vi "XY Graph Get Plot Info & Clip Data.vi"(8 "error in (no error)":errorcluster, 9 "Clip Plot? (True)":bool=TRUE, 10 "Plot index":i32, 11 "XYGraph Ref in":refnum<vi>) -> (0 "error out":errorcluster, 1 "Y Array":dbl[](array[numeric]), 2 "X Array":dbl[](array[numeric]), 3 "XYGraph Ref out":refnum<vi>, 4 "Plot Name":string, 5 "Plot Range":T1, 6 "Plot Color":u32, 7 "Plot Clipped?":bool)   [LabVIEW 2021, in "XY Graph Add-Ons.lvlib"]
doc: "Returns the <B>X</B> and <B>Y</B> array of the selected plot and optionally removes points which are not visible in the <B>XY Graph</B>."
uses:
  XY Graph Add-Ons.lvlib
  Plot Range.ctl
  Graphs.lvlib
panel:
  # "-1: last plot\n-2: next to last plot\n-3: etc..."
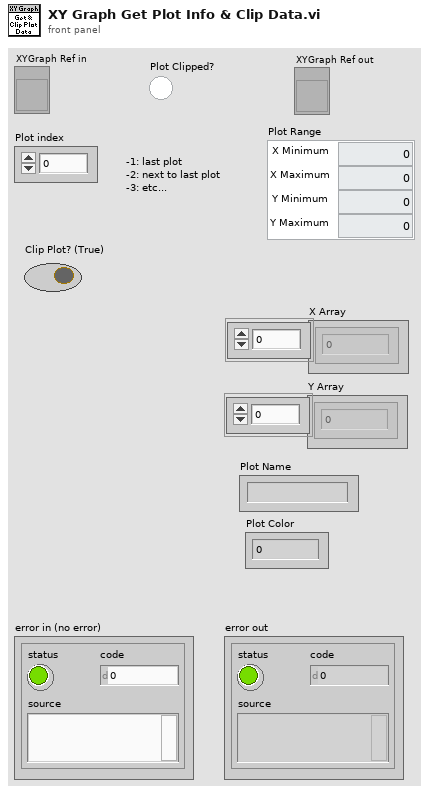
[diagram p1: front panel]
types:
  T1 = typedef "Graphs.lvlib/Plot Range.ctl" = cluster{"X Minimum":dbl, "X Maximum":dbl, "Y Minimum":dbl, "Y Maximum":dbl}
  T2 = cluster{"X Array out":dbl[], "Y Array out":dbl[]}
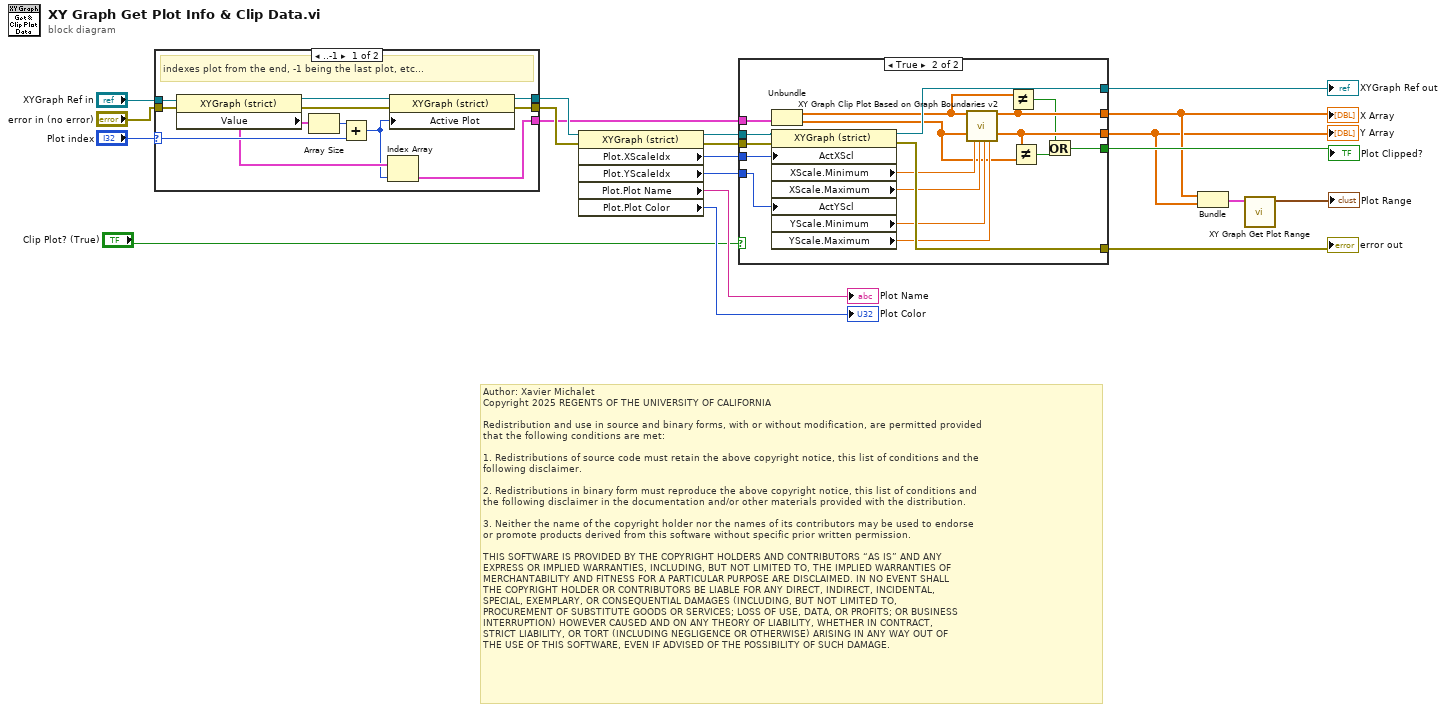
[diagram p0: block diagram]
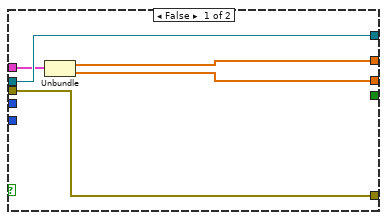
[diagram p2: hidden frame]
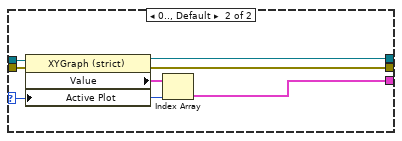
[diagram p3: hidden frame]
diagram:
  # "Author: Xavier Michalet\nCopyright 2025 REGENTS OF THE UNIVERSITY OF CALIFORNIA\n\nRedistribution and use in source and binary forms, with or without modification, are permitted provided\nthat the following conditions are met:\n\n1. Redistributions of source code must retain the above copyright notice, this list of conditions and the\nfollowing disclaimer.\n\n2. Redistributions in binary form must reproduce the above copyright notice, this list of conditions and\nthe following disclaimer in the documentation and/or other materials provided with the distribution.\n\n3. Neither the name of the copyright holder nor the names of its contributors may be used to endorse \nor promote products derived from this software without specific prior written permission.\n\nTHIS SOFTWARE IS PROVIDED BY THE COPYRIGHT HOLDERS AND CONTRIBUTORS “AS IS” AND ANY \nEXPRESS OR IMPLIED WARRANTIES, INCLUDING, BUT NOT LIMITED TO, THE IMPLIED WARRANTIES OF\nMERCHANTABILITY AND FITNESS FOR A PARTICULAR PURPOSE ARE DISCLAIMED. IN NO EVENT SHALL\nTHE COPYRIGHT HOLDER OR CONTRIBUTORS BE LIABLE FOR ANY DIRECT, INDIRECT, INCIDENTAL, \nSPECIAL, EXEMPLARY, OR CONSEQUENTIAL DAMAGES (INCLUDING, BUT NOT LIMITED TO, \nPROCUREMENT OF SUBSTITUTE GOODS OR SERVICES; LOSS OF USE, DATA, OR PROFITS; OR BUSINESS\nINTERRUPTION) HOWEVER CAUSED AND ON ANY THEORY OF LIABILITY, WHETHER IN CONTRACT, \nSTRICT LIABILITY, OR TORT (INCLUDING NEGLIGENCE OR OTHERWISE) ARISING IN ANY WAY OUT OF\nTHE USE OF THIS SOFTWARE, EVEN IF ADVISED OF THE POSSIBILITY OF SUCH DAMAGE."
  n1 = case shown="..-1" "Plot index" {
    selector: "Plot index" -> [w28 w33]
    tunnel: [w25 w37] -> w11
    tunnel: "XYGraph Ref in" -> [w31 w36]
    tunnel: "error in (no error)" -> [w30 w35]
    tunnel: [w24 w34] -> w8
    tunnel: [w21 w32] -> w6
    frame ..-1 {
      # "indexes plot from the end, -1 being the last plot, etc..."
      n2 = property class="XYGraph (strict)"(reference=w31, error in=w30) -> (reference out=w27:refnum<vi>, error out=w26:errorcluster, "Value"=w23:cluster{dbl[], dbl[]}[])
      n3 = Array Size(array=w23) -> (size(s)=w29:i32)
      n4 = Add(x=w29, y=w28) -> (x+y=w22:i32)
      n5 = Index Array(array=w23, index=w22) -> (element=w21:cluster{dbl[], dbl[]})
      n6 = property class="XYGraph (strict)"(reference=w27, error in=w26, "Active Plot"=w22) -> (reference out=w25:refnum<vi>, error out=w24:errorcluster)
    }
    frame 0.., Default {
      n7 = property class="XYGraph (strict)"(reference=w36, error in=w35, "Active Plot"=w33) -> (reference out=w37:refnum<vi>, error out=w34:errorcluster, "Value"=w38:cluster{dbl[], dbl[]}[])
      n8 = Index Array(array=w38, index=w33) -> (element=w32:cluster{dbl[], dbl[]})
    }
  }
  n9 = property class="XYGraph (strict)"(reference=w11, error in=w8) -> (reference out=w17:refnum<vi>, error out=w15:errorcluster, "Plot.XScaleIdx"=w13:u32, "Plot.YScaleIdx"=w12:u32, "Plot.Plot Name"=→"Plot Name":string, "Plot.Plot Color"=→"Plot Color":u32)
  n10 = case shown="True" "Clip Plot? (True)" {
    tunnel: w6 -> [w41 w55]
    tunnel: w17 -> [w43 w61]
    tunnel: [w43 w59] -> w16
    tunnel: w15 -> [w42 w60]
    tunnel: [w42 w58] -> w14
    tunnel: w13 -> [_ w57]
    tunnel: w12 -> [_ w56]
    tunnel: [w40 w50] -> w3
    tunnel: [w39 w48] -> w2
    tunnel: [_ w44] -> w4
    frame False {
      n11 = Unbundle(w41) -> (w40:dbl[], w39:dbl[])
    }
    frame True {
      n12 = Unbundle(w55) -> (w49:dbl[], w47:dbl[])
      n13 = property class="XYGraph (strict)"(reference=w61, error in=w60, "ActXScl"=w57, "ActYScl"=w56) -> (reference out=w59:refnum<vi>, error out=w58:errorcluster, "XScale.Minimum"=w54:dbl, "XScale.Maximum"=w53:dbl, "YScale.Minimum"=w52:dbl, "YScale.Maximum"=w51:dbl)
      n14 = call "XY Graph Clip Plot Based on Graph Boundaries v2.vi"("X Array in"=w49, "Y Array in"=w47, "XScale.Minimum (-Inf)"=w54, "XScale.Maximum (Inf)"=w53, "YScale.Minimum (-Inf)"=w52, "YScale.Maximum (Inf)"=w51) -> ("X Array out"=w50:dbl[], "Y Array out"=w48:dbl[])  [unwired: 12 in]
      n15 = Not Equal?(x=w49, y=w50) -> (x != y?=w45:bool)
      n16 = Not Equal?(x=w48, y=w47) -> (x != y?=w46:bool)
      n17 = Or(x=w45, y=w46) -> (x .or. y?=w44:bool)
    }
  }
  "X Array" <- w3
  "Y Array" <- w2
  "XYGraph Ref out" <- w16
  "error out" <- w14
  "Plot Clipped?" <- w4
  n18 = Bundle("X Array out"=w3, "Y Array out"=w2) -> (w1:T2)  [unwired: 1 in]
  n19 = call "XY Graph Get Plot Range.vi"("Plot in"=w1) -> ("Plot Range"=→"Plot Range":T1)  [unwired: 10 in]
